vi "Get Display String.vi"(11 "Str Equal in":refnum<class "Str Equal.lvclass">) -> (2 "Display String":string)   [LabVIEW 2018, in "Str Equal.lvclass"]
uses:
  Str Equal.lvclass
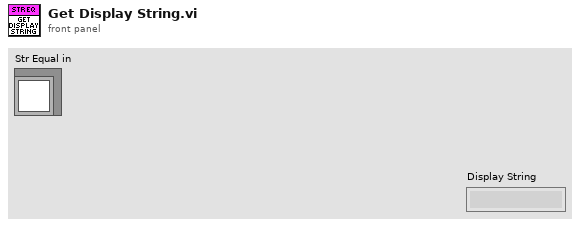
[diagram p1: front panel]
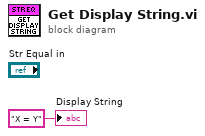
[diagram p0: block diagram]
diagram:
  "Display String" <- "X = Y" ("Display String")
